vi "Write New UI Reference Msg.vi"(10 "Chat Window Model.lvlib:New UI Reference Msg.lvclass":refnum<class "New UI Reference Msg.lvclass">, 11 "Chat Window Model in":refnum<class "Chat Window Model.lvclass">) -> (3 "Chat Window Model out":refnum<class "Chat Window Model.lvclass">)   [LabVIEW 2014, in "Chat Window Model.lvlib" / "Chat Window Model.lvclass"]
uses:
  Chat Window Model.lvclass
  Chat Window Model Messages/New UI Reference Msg/New UI Reference Msg.lvclass
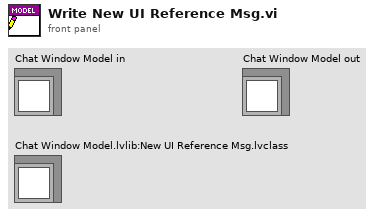
[diagram p1: front panel]
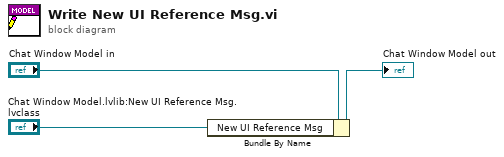
[diagram p0: block diagram]
diagram:
  n1 = Bundle By Name(cluster="Chat Window Model in", "New UI Reference Msg"="Chat Window Model.lvlib:New UI Reference Msg.lvclass") -> (→"Chat Window Model out":refnum<class "Chat Window Model.lvclass">)
